vi "StopLoop.vi"(8 "error in":errorcluster) -> (0 "error out":errorcluster)   [LabVIEW 2009, in "Main.lvlib"]
uses:
  Main.lvlib
  <vilib>/Platform/TimedLoop/XDataNode/XDataNode.xnode
  <vilib>/Platform/TimedLoop/XDataNode/loadlvalarms.vi
  <vilib>/Platform/TimedLoop/XDataNode/timing_clust.ctl
  <vilib>/Platform/TimedLoop/XDataNode/nitl_modes.ctl
  <vilib>/Platform/TimedLoop/XDataNode/wakeup.ctl
  OWNCAN.lvlib
  NetworkVarTarget.lvlib
  <vilib>/Platform/TimedLoop/XDataNode/XDNodeRunTimeDep.lvlib
  MainVariables.lvlib
  Drive.lvlib
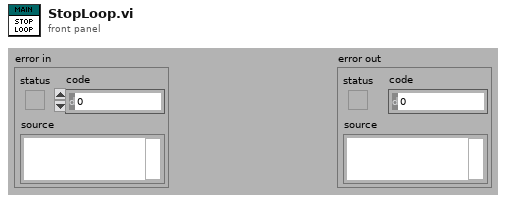
[diagram p1: front panel]
types:
  T1 = typedef "XDNodeRunTimeDep.lvlib/timing_clust.ctl" = cluster{"Expected End [f-1]":u64, "Actual End [f-1]":u64, "Finished Late? [f-1]":bool, "Expected End [i-1]":u64, "Actual End [i-1]":u64, "Finished Late? [i-1]":bool, "Expected Start [i]":u64, "Actual Start [i]":u64, "Expected Start [f]":u64, "Actual Start [f]":u64, "Source Name":string, "Structure Name":string, "Period":i64, "Deadline":i64, "Offset":i64, "Start":i64, "Priority":i32, "Timeout":i32, "Mode":T2, "Wakeup Reason":T3, "Error":errorcluster, "Source Type":string, "Secondary Source Type":string, "Global End Time":u64, "Global Start Time":u64, "Frame Duration":u64, "Iteration Duration":u64, "Assigned CPU":i32, "I/O Scan Engine Mode":u32}
  T2 = typedef "XDNodeRunTimeDep.lvlib/nitl_modes.ctl" = enum32{"No Change", "Process missed periods, maintain original phase", "Discard missed periods, maintain original phase", "Process missed periods, ignore original phase", "Discard missed periods, ignore original phase"}
  T3 = typedef "XDNodeRunTimeDep.lvlib/wakeup.ctl" = enum32{"Normal", "Aborted", "Asynchronous wakeup", "Timing source error", "Timed loop error", "Timeout"}
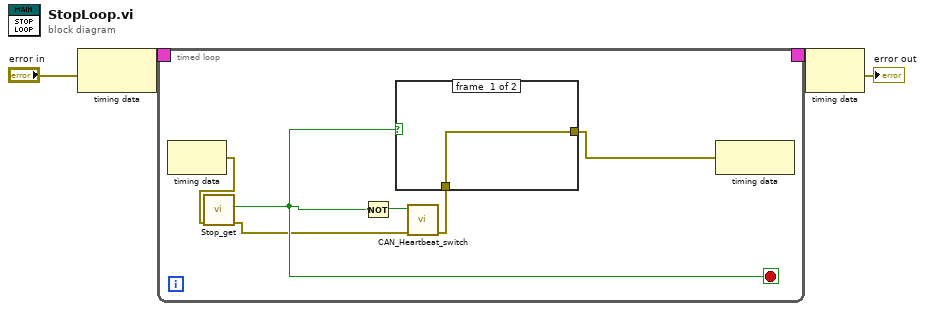
[diagram p0: block diagram]
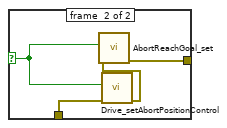
[diagram p2: hidden frame]
diagram:
  n1 = node-c288("error in") -> (w4:T1)
  n2 = timed-loop {
    timing: w4 -> [_]
    timing-out: [_] -> w3
    stop <- w9 stop-if-true
    n3 = node-c288() -> (w8:errorcluster)  [unwired: 1 in]
    n4 = call "Stop_get.vi"("error in (no error)"=w8) -> ("error out"=w7:errorcluster, "Stop"=w9:bool)  [unwired: 9 in]
    n5 = Not(x=w9) -> (.not. x?=w10:bool)
    n6 = call "CAN_Heartbeat_switch.vi"("error in"=w7, "Enable? (T)"=w10) -> ("error out"=w6:errorcluster)  [unwired: 9 in]
    n7 = case shown="False" w9 {
      selector: w9 -> [_ w15]
      tunnel: w6 -> [w11 w14]
      tunnel: [w11 w12] -> w5
      frame #0 {
      }
      frame #1 {
        n8 = call "Drive_setAbortPositionControl.vi"("error in (no error)"=w14, "Abort? (F)"=w15) -> ("error out"=w13:errorcluster)  [unwired: 9 in]
        n9 = call "AbortReachGoal_set.vi"("error in (no error)"=w13, "Abort? (F)"=w15) -> ("error out"=w12:errorcluster)  [unwired: 9 in]
      }
    }
    n10 = node-c288(w5) -> ()  [unwired: 1 out]
  }
  n11 = node-c288(w3) -> (→"error out":errorcluster)
